vi "SolenoidToggle.vi"(0 "Button Press":bool, 9 "x":bool) -> (4 "Boolean":bool)   [LabVIEW 2018]
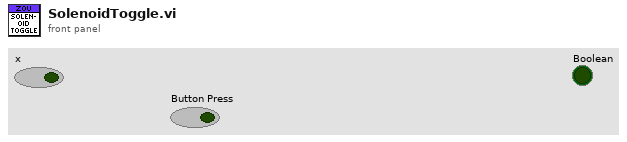
[diagram p1: front panel]
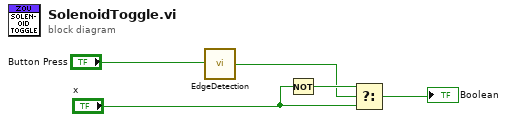
[diagram p0: block diagram]
diagram:
  n1 = call "EdgeDetection.vi"("Boolean"="Button Press") -> ("Boolean 2"=w1:bool)  [unwired: 14 in]
  n2 = Not(x="x") -> (.not. x?=w5:bool)
  n3 = Select(t=w5, s=w1, f="x") -> (s? t:f=→"Boolean":bool)
